vi "Powerup Diagnostics.vi"() -> (0 "error out":errorcluster, 3 "Current":dbl=4.75)   [LabVIEW 2025]
doc: "Performs Diagnostics on the Power Supply unit. Returns the measured current output of the power supply."
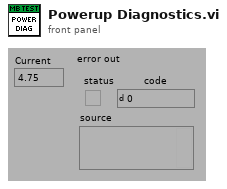
[diagram p1: front panel]
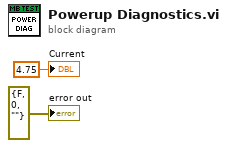
[diagram p0: block diagram]
diagram:
  "error out" <- errorcluster {"status"=FALSE, "code"=0, "source"=""} ("error out")
  "Current" <- 4.75 ("Numeric Measurement")
